vi "Receive Shortcut Menu Selection Event.vi"(8 "error in (no error)":errorcluster, 10 "ShortcutMenuSelectionMsg":refnum<class "ShortcutMenuSelectionMsg.lvclass">, 11 "Test Executive Builder View In":refnum<class "Test Executive Builder View.lvclass">) -> (0 "error out":errorcluster, 3 "Test Executive Builder View Out":refnum<class "Test Executive Builder View.lvclass">)   [LabVIEW 2017, in "Test Executive Builder View.lvclass"]
doc: "<License>\nCopyright © 2017 Composed Systems, LLC | All rights reserved\nwww.composed.io\n\nAuthor: Ethan Stern <ethan.stern@composed.io>\n\nThis software is provided \"AS IS\" WITHOUT WARRANTIES, either express or implied, AND IS FOR EDUCATIONAL PURPOSES ONLY.\n</License>"
uses:
  Test Executive Builder View.lvclass
  <vilib>/gpm_packages/@cs/mva-viewable/Source/ActorEvents/IEventAggregator Messages/ShortcutMenuSelectionMsg/ShortcutMenuSelectionMsg.lvclass
  <vilib>/gpm_packages/@cs/mva-viewable/Source/ActorEvents/IEventAggregator Messages/ShortcutMenuSelectionMsg/ShortcutMenuSelectionMsg.lvclass/ShortcutMenuSelectionMsg.ctl
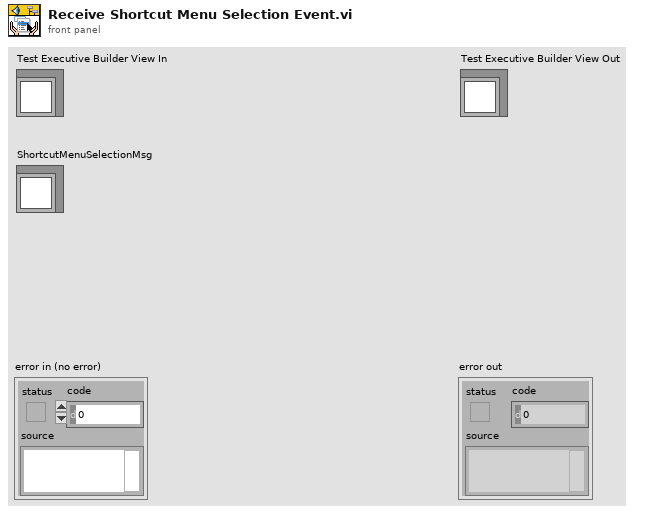
[diagram p1: front panel]
types:
  T1 = typedef "LVPoint32TypeDef.ctl" = cluster{"Horizontal":i32, "Vertical":i32}
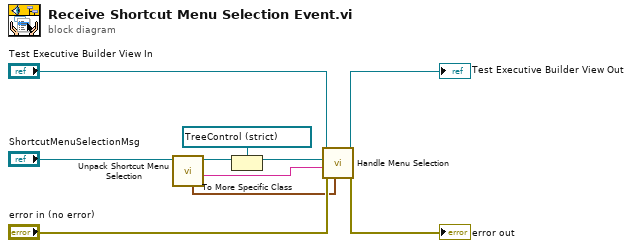
[diagram p0: block diagram]
diagram:
  n1 = call <vilib>:"Unpack Shortcut Menu Selection.vi"("ShortcutMenuSelectionMsg"="ShortcutMenuSelectionMsg") -> ("Item Tag"=w2:string, "CtlRef"=w9:refnum<vi>, "Coords"=w1:T1)  [unwired: 3 in, 5 out]
  n2 = To More Specific Class(target class=refnum<vi> refnum ("Tree Ref"), reference=w9) -> (specific class reference=w3:refnum<vi>)  [unwired: 1 in, 1 out]
  n3 = call-dynamic "Handle Menu Selection.vi"("Coords"=w1, "error in (no error)"="error in (no error)", "Item Tag"=w2, "Tree Refnum"=w3, "Test Executive Builder View in"="Test Executive Builder View In") -> ("error out"=→"error out":errorcluster, "Test Executive Builder View out"=→"Test Executive Builder View Out":refnum<class "Test Executive Builder View.lvclass">)  [unwired: 5 in]
